vi "InitializeRequest.vi"(8 "error in (no error)":errorcluster, 9 "Reset":bool, 10 "IDQuery":bool, 11 "ModuleID":i32) -> (0 "error out":errorcluster)   [LabVIEW 2018, in "FgenPlugins.lvlib" / "FgenPluginsBase.lvclass"]
uses:
  FgenPluginsBase.lvclass
  FgenModule/Protected/clEventType.ctl
  TypeDefs/InitOptions.ctl
  <vilib>/Utility/error.llb/Error Cluster From Error Code.vi
  <vilib>/ErrorRing/Error Ring.xnode
  FgenModule/FgenModule.lvlib
  FgenPlugins.lvlib
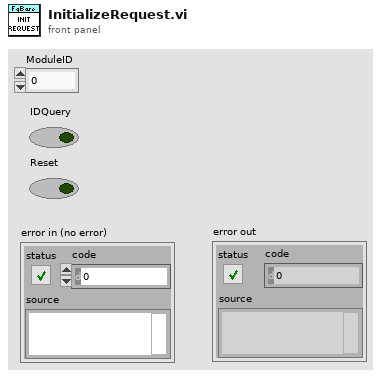
[diagram p1: front panel]
types:
  T1 = typedef "FgenModule.lvlib/clRequestEvents.ctl" = cluster{"StopRequest":refnum<user-event>, "PathToINI":refnum<user-event>, " LoadPlugin":refnum<user-event>, "ShowPanel":refnum<user-event>, "Initialize":refnum<user-event>, "GetChannels":refnum<user-event>, "SetChannels":refnum<user-event>, "Abort":refnum<user-event>, "Initiate":refnum<user-event>, "ConfigDlg":refnum<user-event>, "GetFunction":refnum<user-event>, "SetFunction":refnum<user-event>, "ConfigFunction":refnum<user-event>, "GetWfrm":refnum<user-event>, "SetWfrm":refnum<user-event>, "GetTriggers":refnum<user-event>, "SetTriggers":refnum<user-event>, "ConfigTriggers":refnum<user-event>}
  T2 = typedef "FgenPlugins.lvlib/InitOptions.ctl" = cluster{"IDQuery":bool, "Reset":bool}
  T3 = typedef "FgenModule.lvlib/clEventType.ctl" = cluster{"ModuleID":i32, "Data":variant}
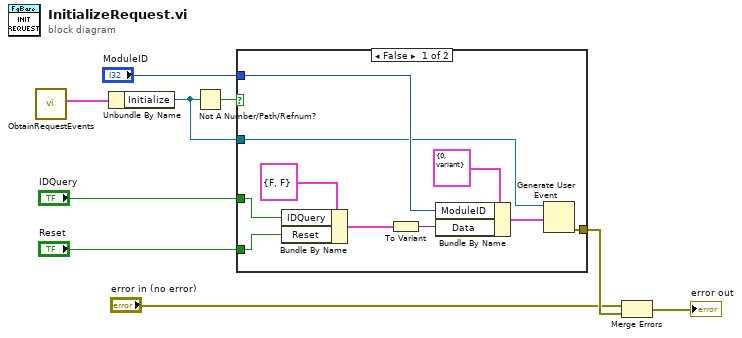
[diagram p0: block diagram]
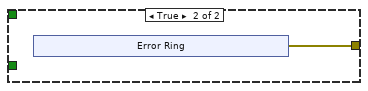
[diagram p2: hidden frame]
diagram:
  n1 = call "ObtainRequestEvents.vi"() -> ("clRequestEvents"=w9:T1)  [unwired: 10 in, 1 out]
  n2 = Unbundle By Name(w9) -> ("Initialize"=w7:refnum<user-event>)
  n3 = Not A Number/Path/Refnum?(number/path/refnum=w7) -> (NaN/Path/Refnum?=w8:bool)
  n4 = case shown="False" w8 {
    tunnel: w7 -> [w16 _]
    tunnel: "ModuleID" -> [w18 _]
    tunnel: [w15 w20] -> w4
    tunnel: "IDQuery" -> [w12 _]
    tunnel: "Reset" -> [w11 _]
    frame False {
      n5 = Bundle By Name(cluster=T2 {"IDQuery"=FALSE, "Reset"=FALSE} ("InitOptions"), "IDQuery"=w12, "Reset"=w11) -> (w13:T2)
      n6 = To Variant(anything=w13) -> (Variant=w14:variant)
      n7 = Bundle By Name(cluster=T3 {"ModuleID"=0, "Data"=variant} ("clEventType"), "ModuleID"=w18, "Data"=w14) -> (w17:T3)
      n8 = Generate User Event(user event=w16, event data cluster=w17) -> (error out=w15:errorcluster)  [unwired: 2 in, 1 out]
    }
    frame True {
      n9 = xnode "Error Ring"() -> ("error out"=w20:errorcluster)
    }
  }
  n10 = Merge Errors("error in (no error)", w4) -> (→"error out":errorcluster)
